vi "Write SetRequest.vi"(5 "Timeout (-1)":i32=-1, 7 "Synchronous (F)":bool, 8 "error in (no error)":errorcluster, 10 "Value":variant, 11 "Tag in":refnum<class "Tag.lvclass">) -> (0 "error out":errorcluster, 2 "timed out?":bool, 3 "Tag out":refnum<class "Tag.lvclass">)   [LabVIEW 2018, in "Tag Engine.lvlib" / "Tag.lvclass"]
doc: "_SubVI_"
uses:
  Tag.lvclass
  Tag.lvclass/Tag.ctl
  Types/SetRequest Cluster.ctl
  <vilib>/Utility/Data Type/Type Definitions/Data Type.ctl
  Tag Engine.lvlib
  <vilib>/Utility/Data Type/NI_Data Type.lvlib
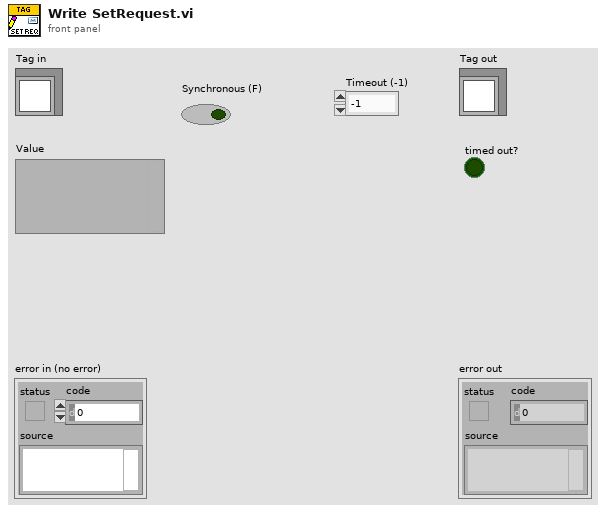
[diagram p1: front panel]
types:
  T1 = typedef "Tag Engine.lvlib/SetRequest Cluster.ctl" = cluster{"Tag Name":string, "Type":T2, "Old Value":variant, "Old Time Stamp":timestamp, "Req Value":variant, "Req Time Stamp":timestamp, "Callback":refnum<notifier>, "Synchronous (F)":bool}
  T2 = typedef "NI_Data Type.lvlib/Data Type.ctl" = enum8{"Invalid Type", "Void", "I8", "I16", "I32", "I64", "U8", "U16", "U32", "U64", "Single Float", "Double Float", "Extended Float", "Single Complex", "Double Complex", "Extended Complex", "Enum U8", "Enum U16", "Enum U32", "Enum U64", "Single Float With Unit", "Double Float With Unit", "Extended Float With Unit", "Single Complex with Unit", "Double Complex with Unit", "Extended Complex with Unit", "Boolean", "String", "Path", "Picture", "Tag", "Array", "Cluster", "Variant", "LV Variant", "Waveform", "Timestamp", "Digital Waveform", "Digital Data", "ExpressData", "Refnum", "External Data", "VI", "Poly VI", "LabVIEW Class Instance", "Fixed Point"}
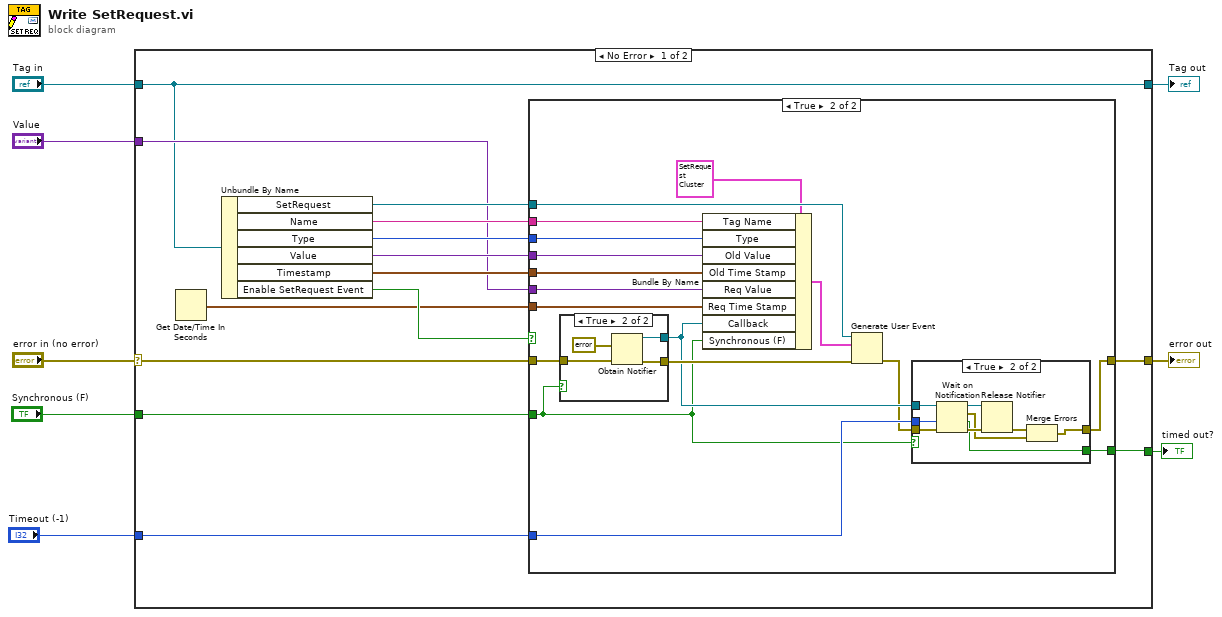
[diagram p0: block diagram]
diagram:
  n1 = case shown="No Error" "error in (no error)" {
    selector: "error in (no error)" -> [w12 w56]
    tunnel: [w18 w56] -> w7
    tunnel: [w13 w57] -> w5
    tunnel: "Tag in" -> [w13 w57]
    tunnel: "Value" -> [w15 _]
    tunnel: "Synchronous (F)" -> [w11 _]
    tunnel: "Timeout (-1)" -> [w10 _]
    tunnel: [w9 _] -> w1
    frame No Error {
      n2 = Get Date/Time In Seconds() -> (seconds since 1Jan1904=w14:timestamp)
      n3 = Unbundle By Name(w13) -> ("SetRequest"=w19:refnum<user-event>, "Name"=w21:string, "Type"=w20:T2, "Value"=w17:variant, "Timestamp"=w16:timestamp, "Enable SetRequest Event"=w22:bool)
      n4 = case shown="True" w22 {
        tunnel: w21 -> [_ w38]
        tunnel: w20 -> [_ w37]
        tunnel: w19 -> [_ w40]
        tunnel: w12 -> [w23 w31]
        tunnel: [w23 w25] -> w18
        tunnel: w17 -> [_ w36]
        tunnel: w16 -> [_ w35]
        tunnel: w15 -> [_ w34]
        tunnel: w14 -> [_ w33]
        tunnel: w11 -> [_ w26]
        tunnel: w10 -> [_ w28]
        tunnel: [_ w24] -> w9
        frame False {
        }
        frame True {
          n5 = case shown="True" w26 {
            tunnel: w31 -> [w51 w54]
            tunnel: [_ w53] -> w29
            tunnel: [w51 w52] -> w30
            frame False {
            }
            frame True {
              n6 = Obtain Notifier(notification data type=errorcluster {"status"=FALSE, "code"=0, "source"=""} ("error in (no error)"), error in (no error)=w54) -> (notifier out=w53:refnum<notifier>, error out=w52:errorcluster)  [unwired: 2 in, 1 out]
            }
          }
          n7 = Bundle By Name(cluster=T1 {"Tag Name"="", "Type"=enum."Variant", "Old Value"=variant, "Old Time Stamp"=timestamp(0 s since 1904-01-01), "Req Value"=variant, "Req Time Stamp"=timestamp(0 s since 1904-01-01), "Callback"=refnum, "Synchronous (F)"=FALSE} ("event data"), "Tag Name"=w38, "Type"=w37, "Old Value"=w36, "Old Time Stamp"=w35, "Req Value"=w34, "Req Time Stamp"=w33, "Callback"=w29, "Synchronous (F)"=w26) -> (w32:T1)
          n8 = Generate User Event(user event=w40, event data cluster=w32, error in=w30) -> (error out=w27:errorcluster)  [unwired: 1 in, 1 out]
          n9 = case shown="True" w26 {
            tunnel: w29 -> [_ w50]
            tunnel: w28 -> [_ w49]
            tunnel: w27 -> [w41 w48]
            tunnel: [w41 w43] -> w25
            tunnel: [_ w42] -> w24
            frame False {
            }
            frame True {
              n10 = Wait on Notification(notifier=w50, timeout in ms (-1)=w49, error in (no error)=w48) -> (notifier out=w46:refnum<notifier>, notification=w44:errorcluster, timed out?=w42:bool, error out=w47:errorcluster)  [unwired: 1 in]
              n11 = Release Notifier(notifier=w46, error in (no error)=w47) -> (error out=w45:errorcluster)  [unwired: 1 in, 2 out]
              n12 = Merge Errors(w45, w44) -> (w43:errorcluster)
            }
          }
        }
      }
    }
    frame Error {
    }
  }
  "error out" <- w7
  "Tag out" <- w5
  "timed out?" <- w1
